vi "3-5.vi"(1 "X":dbl) -> (0 "Y":dbl)   [LabVIEW 2017]
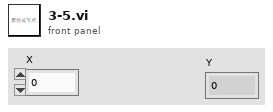
[diagram p1: front panel]
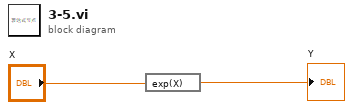
[diagram p0: block diagram]
diagram:
  n1 = expression code="exp(X)"("X") -> (→"Y":dbl)
